vi "移位寄存器初始化.vi"(11 "终端节点数量":dbl) -> (3 "数组":dbl[](array[numeric]))   [LabVIEW 2018]
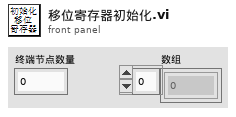
[diagram p1: front panel]
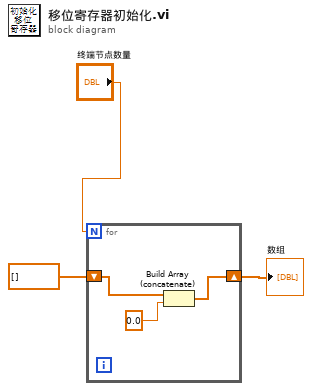
[diagram p0: block diagram]
diagram:
  n1 = for {
    N: "终端节点数量" -> [_]
    shift-right: [w5] -> w2
    shift-left: dbl[] [] -> [w6]
    n2 = Build Array (concatenate)(w6, 0.0 ("数值")) -> (w5:dbl[])
  }
  "数组" <- w2
